vi "Publish Driver Revisions.vi"(8 "error in (no error)":errorcluster, 11 "CS++DeviceActor in":refnum<class "CS++DeviceActor.lvclass">) -> (0 "error out":errorcluster, 3 "CS++DeviceActor out":refnum<class "CS++DeviceActor.lvclass">)   [LabVIEW 2013, in "CS++DeviceActor.lvlib" / "CS++DeviceActor.lvclass"]
doc: "Publish driver revisions."
uses:
  CS++DeviceActor.lvclass
  Classes/CS++ProcessVariables/ProcessVariable/PV.lvclass
  CS++DeviceActor.lvclass/CS++DeviceActor.ctl
  Classes/CS++ProcessVariables/PVConnection/PVConnection.lvclass
  Classes/CS++ProcessVariables/ProcessVariable/PV.lvclass/PV.ctl
  Classes/CS++ProcessVariables/ProcessVariable/Write Data.vi
  Classes/CS++ProcessVariables/ProcessVariable/Write Timestamp.vi
  Classes/CS++ProcessVariables/ProcessVariable/Write Quality.vi
  Classes/CS++ProcessVariables/ProcessVariable/Write status.vi
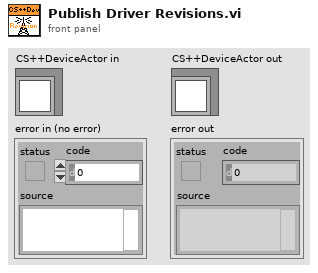
[diagram p1: front panel]
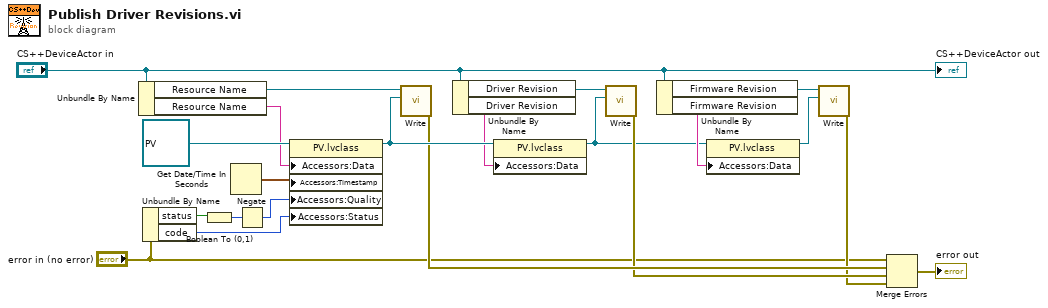
[diagram p0: block diagram]
diagram:
  n1 = Unbundle By Name("CS++DeviceActor in") -> ("Resource Name"=w21:refnum<class "PVConnection.lvclass">, "Resource Name"=w19:string)
  n2 = Unbundle By Name("error in (no error)") -> ("status"=w17:bool, "code"=w14:i32)
  n3 = Boolean To (0,1)(Boolean=w17) -> (0, 1=w16:i16)
  n4 = Get Date/Time In Seconds() -> (seconds since 1Jan1904=w18:timestamp)
  n5 = Negate(x=w16) -> (-x=w15:i16)
  n6 = property class="PV.lvclass"(reference=refnum<class "PV.lvclass"> refnum ("CS++ProcessVariables.lvlib:PV.lvclass"), "Accessors:Data"=w19, "Accessors:Timestamp"=w18, "Accessors:Quality"=w15, "Accessors:Status"=w14) -> (reference out=w12:refnum<class "PV.lvclass">)  [unwired: 1 in, 1 out]
  n7 = call-dynamic "Write.vi"("PV"=w12, "PVConnection in"=w21) -> ("error out"=w6:errorcluster)  [unwired: 8 in, 1 out]
  n8 = Unbundle By Name("CS++DeviceActor in") -> ("Driver Revision"=w13:refnum<class "PVConnection.lvclass">, "Driver Revision"=w11:string)
  n9 = property class="PV.lvclass"(reference=w12, "Accessors:Data"=w11) -> (reference out=w1:refnum<class "PV.lvclass">)  [unwired: 1 in, 1 out]
  n10 = call-dynamic "Write.vi"("PV"=w1, "PVConnection in"=w13) -> ("error out"=w5:errorcluster)  [unwired: 8 in, 1 out]
  n11 = Unbundle By Name("CS++DeviceActor in") -> ("Firmware Revision"=w9:refnum<class "PVConnection.lvclass">, "Firmware Revision"=w10:string)
  n12 = property class="PV.lvclass"(reference=w1, "Accessors:Data"=w10) -> (reference out=w8:refnum<class "PV.lvclass">)  [unwired: 1 in, 1 out]
  n13 = call-dynamic "Write.vi"("PV"=w8, "PVConnection in"=w9) -> ("error out"=w4:errorcluster)  [unwired: 8 in, 1 out]
  n14 = Merge Errors("error in (no error)", w6, w5, w4) -> (→"error out":errorcluster)
  "CS++DeviceActor out" <- "CS++DeviceActor in"
